vi "Envelope.vi"(4 "Waveform":dbl[](array[numeric]), 5 "Hilbert Transform/Clip Method":bool) -> (1 "Envelope":dbl[](array[numeric]))   [LabVIEW 2013]
uses:
  <vilib>/measure/mascope.llb/Amplitude and Levels 1 chan.vi
  <vilib>/Analysis/NI_AALPro.lvlib
  <vilib>/measure/NI_MAPro.lvlib
panel:
  out "Waveform Graph":dbl[][](graph)
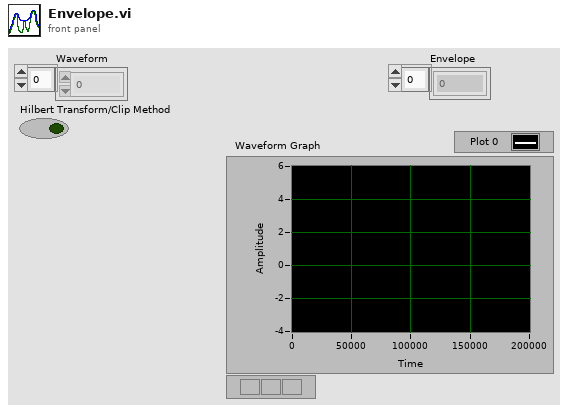
[diagram p1: front panel]
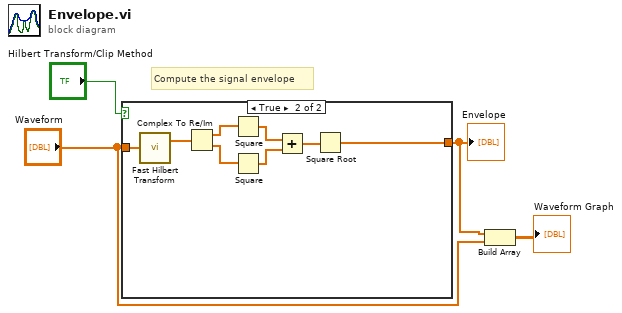
[diagram p0: block diagram]
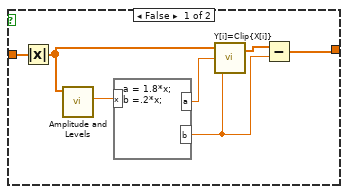
[diagram p2: hidden frame]
diagram:
  # "Compute the signal envelope"
  n1 = case shown="True" "Hilbert Transform/Clip Method" {
    tunnel: "Waveform" -> [w11 w19]
    tunnel: [w5 w12] -> w2
    frame False {
      n2 = Absolute Value(x=w11) -> (abs(x)=w10:dbl[])
      n3 = call-poly <vilib>:"Amplitude and Levels.vi"("signal in"=w10) -> ("high state level"=w8:dbl)  [unwired: 7 in, 3 out]
      n4 = formula code="a = 1.8*x;\nb =.2*x;"("x"=w8) -> ("a"=w9:dbl, "b"=w6:dbl)
      n5 = call <vilib>:"Y[i]=Clip{X[i]}.vi"("lower limit"=w6, "upper limit"=w9, "Input Array"=w10) -> ("Clipped Array"=w7:dbl[])  [unwired: 1 out]
      n6 = Subtract(x=w7, y=w6) -> (x-y=w5:dbl[])
    }
    frame True {
      n7 = call <vilib>:"Fast Hilbert Transform.vi"("X"=w19) -> ("Hilbert{X}"=w13:dbl[])  [unwired: 1 out]
      n8 = Complex To Re/Im(x + iy=w13) -> (x=w18:dbl[], y=w17:dbl[])
      n9 = Square(x=w18) -> (x^2=w16:dbl[])
      n10 = Square(x=w17) -> (x^2=w15:dbl[])
      n11 = Add(x=w16, y=w15) -> (x+y=w14:dbl[])
      n12 = Square Root(x=w14) -> (sqrt(x)=w12:dbl[])
    }
  }
  "Envelope" <- w2
  n13 = Build Array(w2, "Waveform") -> (→"Waveform Graph":dbl[][])
